vi "scanObjToTxt.vi"(3 "error in (no error)":errorcluster, 4 "Path":path, 5 "Scan":refnum<class "Scan.lvclass">) -> (0 "error out":errorcluster)   [LabVIEW 2017]
uses:
  classes/Scans/Scan.lvclass
  classes/Scans/Scan.lvclass/Scan.ctl
  classes/Scans/Read A scans.vi
  classes/Scans/Read B scans.vi
  classes/Scans/Read C scans.vi
  classes/Scans/Read Repeat B scans.vi
  classes/Scans/Read Scan Angle (degrees).vi
  classes/Scans/Read X FOV (degrees).vi
  classes/Scans/Read X offset (degrees).vi
  classes/Scans/Read Y FOV (degrees).vi
  classes/Scans/Read Y offset (degrees).vi
  classes/Scans/Read Bidirectional.vi
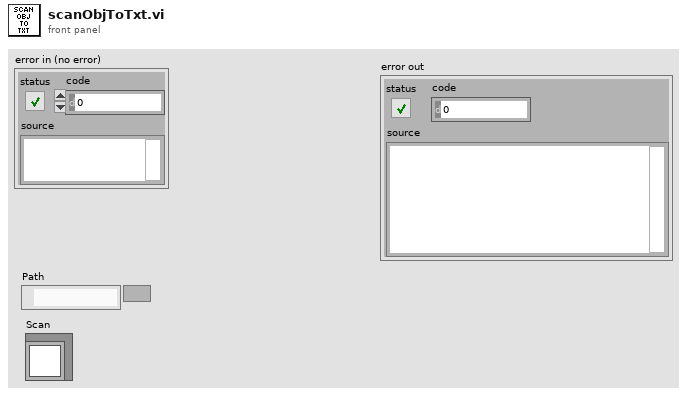
[diagram p1: front panel]
types:
  T1 = enum16{"open", "replace", "create", "open or create", "replace or create", "replace or create with confirmation"}
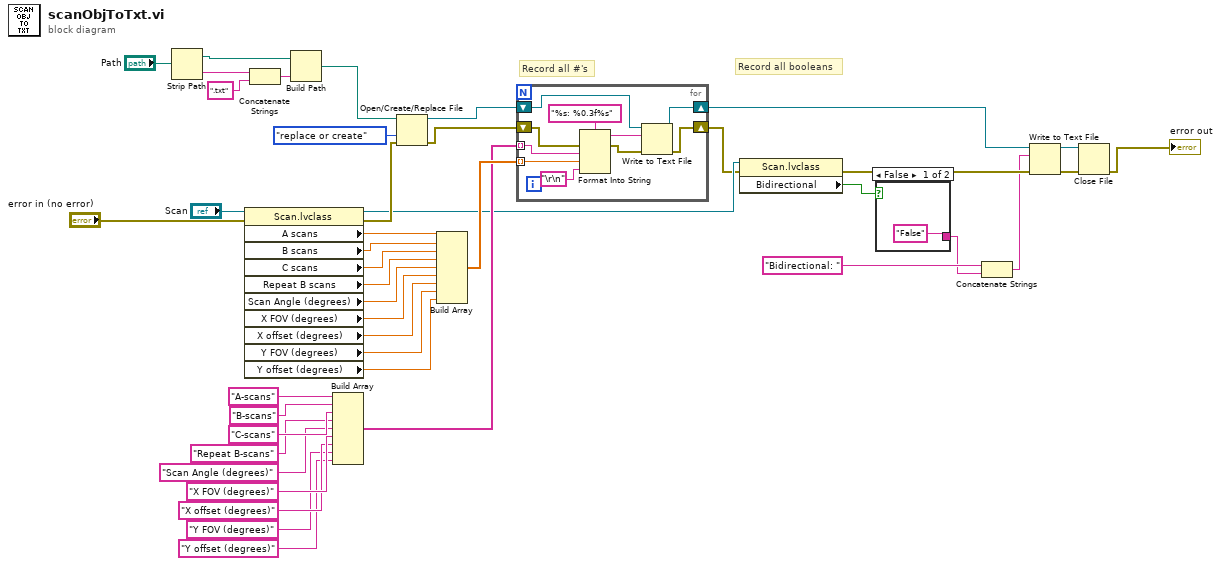
[diagram p0: block diagram]
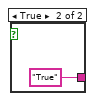
[diagram p2: hidden frame]
diagram:
  # "Record all booleans"
  # "Record all #'s"
  n1 = Strip Path(path="Path") -> (stripped path=w5:path, name=w7:string)
  n2 = property class="Scan.lvclass"(reference="Scan", error in="error in (no error)") -> (reference out=w17:refnum<class "Scan.lvclass">, error out=w40:errorcluster, "A scans"=w22:dbl, "B scans"=w23:dbl, "C scans"=w24:dbl, "Repeat B scans"=w25:dbl, "Scan Angle (degrees)"=w26:dbl, "X FOV (degrees)"=w27:dbl, "X offset (degrees)"=w28:dbl, "Y FOV (degrees)"=w29:dbl, "Y offset (degrees)"=w30:dbl)
  n3 = Concatenate Strings(w7, ".txt" ("name or relative path")) -> (w4:string)
  n4 = Build Path(base path=w5, name or relative path=w4) -> (appended path=w42:path)
  n5 = Build Array("A-scans" ("initial string"), "B-scans" ("initial string"), "C-scans" ("initial string"), "Repeat B-scans" ("initial string"), "Scan Angle (degrees)" ("initial string"), "X FOV (degrees)" ("initial string"), "X offset (degrees)" ("initial string"), "Y FOV (degrees)" ("initial string"), "Y offset (degrees)" ("initial string")) -> (w20:string[])
  n6 = Open/Create/Replace File(file path (use dialog)=w42, error in=w40, operation (0:open)=T1."replace or create") -> (refnum out=w19:refnum<file>, error out=w18:errorcluster)  [unwired: 3 in, 1 out]
  n7 = Build Array(w22, w23, w24, w25, w26, w27, w28, w29, w30) -> (w21:dbl[])
  n8 = for {
    tunnel: w21 -> [w52] mode=indexing
    tunnel: w20 -> [w53] mode=indexing
    shift-right: [w46] -> w13
    shift-left: w19 -> [w48]
    shift-right: [w45] -> w9
    shift-left: w18 -> [w49]
    n9 = Format Into String(format string="%s: %0.3f%s", error in=w49, w53, w52, "\r\n") -> (resulting string=w50:string, error out=w47:errorcluster)  [unwired: 1 in]
    n10 = Write to Text File(file (use dialog)=w48, text=w50, error in=w47) -> (refnum out=w46:refnum<file>, error out=w45:errorcluster)  [unwired: 1 in, 1 out]
  }
  n11 = property class="Scan.lvclass"(reference=w17, error in=w9) -> (error out=w11:errorcluster, "Bidirectional"=w16:bool)  [unwired: 1 out]
  n12 = case shown="False" w16 {
    tunnel: ["False" ("initial string") "True" ("initial string")] -> w14
    frame False {
    }
    frame True {
    }
  }
  n13 = Concatenate Strings("Bidirectional: " ("initial string"), w14) -> (w10:string)
  n14 = Write to Text File(file (use dialog)=w13, text=w10, error in=w11) -> (refnum out=w12:refnum<file>, error out=w8:errorcluster)  [unwired: 1 in, 1 out]
  n15 = Close File(refnum=w12, error in=w8) -> (error out=→"error out":errorcluster)  [unwired: 1 out]
